vi "Set Tuner Gain Mode.vi"(8 "error in (no error)":errorcluster, 10 "AutoGain":bool, 11 "RTL-SDR in":refnum<class "RTL-SDR.lvclass">) -> (0 "error out":errorcluster, 1 "function return":i32, 3 "RTL-SDR out":refnum<class "RTL-SDR.lvclass">)   [LabVIEW 2015, in "RTL-SDR.lvclass"]
uses:
  RTL-SDR.lvclass
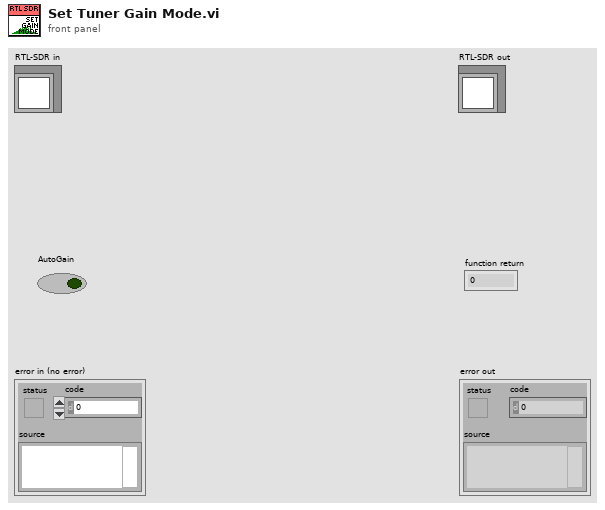
[diagram p1: front panel]
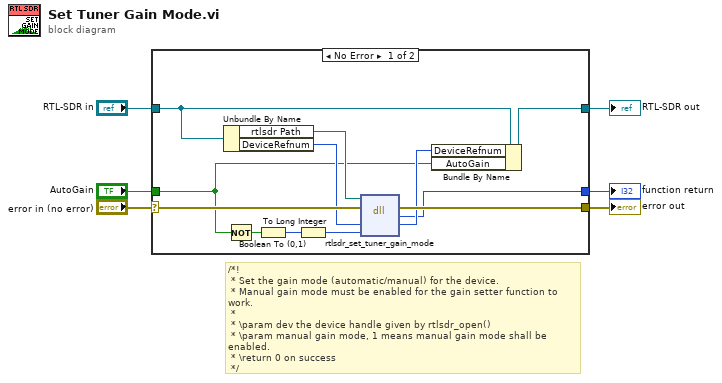
[diagram p0: block diagram]
diagram:
  # "/*!\n * Set the gain mode (automatic/manual) for the device.\n * Manual gain mode must be enabled for the gain setter function to work.\n *\n * \\param dev the device handle given by rtlsdr_open()\n * \\param manual gain mode, 1 means manual gain mode shall be enabled.\n * \\return 0 on success\n */\n\n\nRTLSDR_API int rtlsdr_set_tuner_gain_mode(rtlsdr_dev_t *dev, int manual);"
  n1 = case shown="No Error" "error in (no error)" {
    selector: "error in (no error)" -> [w18 w20]
    tunnel: [w17 w20] -> w5
    tunnel: [w13 w19] -> w3
    tunnel: "RTL-SDR in" -> [w16 w19]
    tunnel: [w11 _] -> w2
    tunnel: "AutoGain" -> [w7 _]
    frame No Error {
      n2 = Unbundle By Name(w16) -> ("rtlsdr Path"=w15:path, "DeviceRefnum"=w14:u64)
      n3 = Not(x=w7) -> (.not. x?=w9:bool)
      n4 = Boolean To (0,1)(Boolean=w9) -> (0, 1=w10:i16)
      n5 = To Long Integer(number=w10) -> (32bit integer=w8:i32)
      n6 = dll-call lib="C:/Users/Ivan/Desktop/D-23-09-24 (RTL-SDR)/Project (Pelleng-SDR)/rtlsdr/dll/rtlsdr.*" fn="rtlsdr_set_tuner_gain_mode"(path in=w15, error in=w18, "DeviceRefnum"=w14, "GainMode"=w8) -> (error out=w17:errorcluster, "return type"=w11:i32, "DeviceRefnum"=w12:u64)  [unwired: 2 in, 1 out]
      n7 = Bundle By Name(cluster=w16, "DeviceRefnum"=w12, "AutoGain"=w7) -> (w13:refnum<class "RTL-SDR.lvclass">)
    }
    frame Error {
    }
  }
  "error out" <- w5
  "RTL-SDR out" <- w3
  "function return" <- w2
